vi "SerialComSub.vi"(4 "stop":bool, 6 "input cluster":T1, 7 "state":i64, 9 "Send":bool, 10 "Bool Refnum":refnum<vi>, 11 "VISA Refnum in":refnum<visa-resource-name>) -> (1 "read buffer":string, 2 "return count":u32, 3 "Send return count":u32)   [LabVIEW 2022 SP3]
uses:
  <vilib>/Instr/_visa.llb/VISA Configure Serial Port (Instr).vi
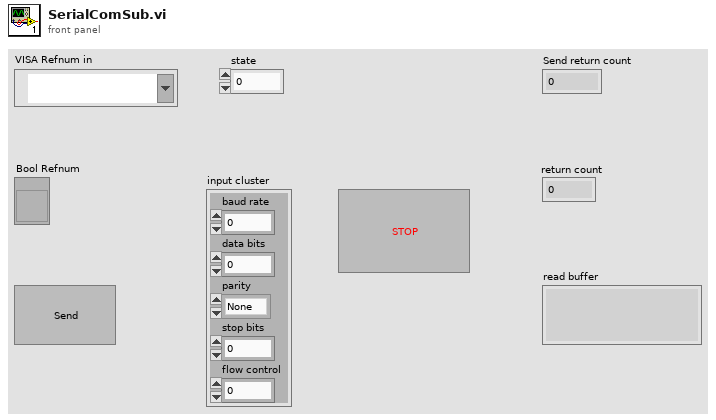
[diagram p1: front panel]
types:
  T1 = cluster{"baud rate":u32, "data bits":u16, "parity":enum16{"None", "Odd", "Even", "Mark", "Space"}, "stop bits":u16, "flow control":u16}
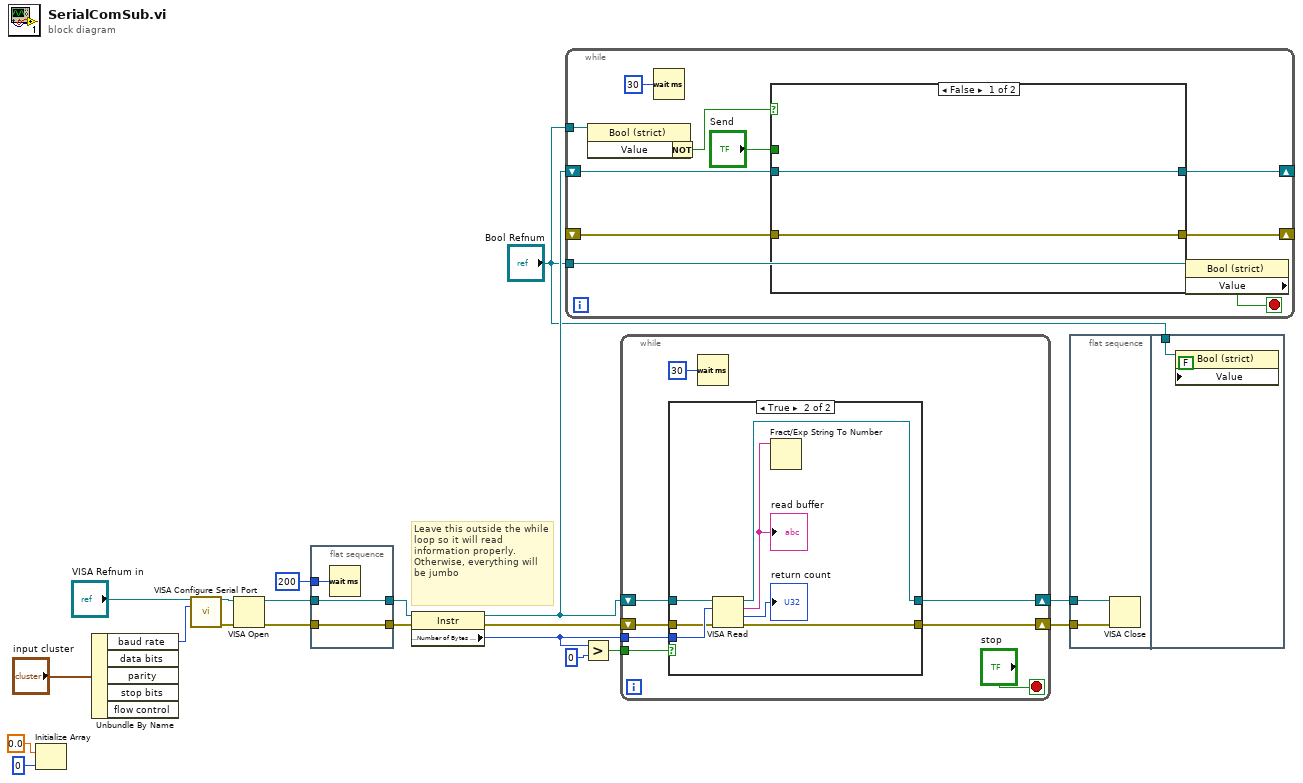
[diagram p0: block diagram]
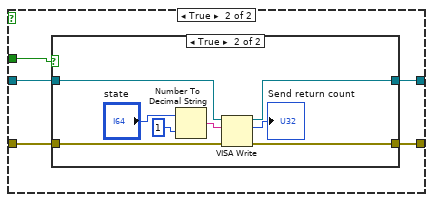
[diagram p2: hidden frame]
diagram:
  # "Leave this outside the while loop so it will read information properly. Otherwise, everything will be jumbo"
  n1 = Initialize Array(0.0, 0) -> ()  [unwired: 1 out]
  n2 = Unbundle By Name("input cluster") -> ("baud rate"=w16:u32)  [unwired: 4 out]
  n3 = call-poly "VISA Configure Serial Port"("VISA resource name"="VISA Refnum in", "baud rate (9600)"=w16) -> ("VISA resource name out"=w18:refnum<visa-resource-name>, "error out"=w19:errorcluster)  [unwired: 12 in]
  n4 = VISA Open(error in (no error)=w19, VISA resource name=w18) -> (VISA resource name=w3:refnum<visa-resource-name>, error out=w4:errorcluster)  [unwired: 3 in]
  n5 = flat-sequence {
    tunnel: w4 -> [w22]
    tunnel: [w22] -> w20
    tunnel: w3 -> [w21]
    tunnel: [w21] -> w7
    tunnel: u32 200 -> [w23]
    frame #0 {
      n6 = Wait (ms)(milliseconds to wait=w23) -> ()  [unwired: 1 out]
    }
  }
  n7 = property class="Instr"(reference=w7, error in=w20) -> (reference out=w9:refnum<visa-resource-name>, error out=w11:errorcluster, "Serial Settings:Number of Bytes at Serial Port"=w10:u32)
  n8 = while {
    shift-right: [w33] -> _
    shift-left: w9 -> [w34]
    shift-right: [w30] -> _
    shift-left: _ -> [w31]
    tunnel: "Bool Refnum" -> [w25]
    tunnel: "Bool Refnum" -> [w24]
    stop <- w29 stop-if-true
    n9 = property on="Property Node" class="Bool (strict)"(reference=w24) -> ("Value"=w28:bool)  [unwired: 1 in, 2 out]
    n10 = Wait (ms)(milliseconds to wait=u32 30) -> ()  [unwired: 1 out]
    n11 = Not(x=w28) -> (.not. x?=w27:bool)
    n12 = case shown="False" w27 {
      tunnel: w34 -> [w36 w40]
      tunnel: [w36 w37] -> w33
      tunnel: w31 -> [w35 w39]
      tunnel: [w35 w38] -> w30
      tunnel: "Send" -> [_ w41]
      frame False {
      }
      frame True {
        n13 = case shown="True" w41 {
          tunnel: w40 -> [w43 w47]
          tunnel: w39 -> [w42 w46]
          tunnel: [w42 w44] -> w38
          tunnel: [w43 w45] -> w37
          frame False {
          }
          frame True {
            n14 = Number To Decimal String(number="state", width (-)=i16 1) -> (decimal integer string=w50:string)
            n15 = VISA Write(VISA resource name=w47, write buffer=w50, error in (no error)=w46) -> (VISA resource name out=w45:refnum<visa-resource-name>, return count=→"Send return count":u32, error out=w44:errorcluster)
          }
        }
      }
    }
    n16 = property on="Property Node" class="Bool (strict)"(reference=w25) -> ("Value"=w29:bool)  [unwired: 1 in, 2 out]
  }
  n17 = Greater?(x=w10, y=u32 0) -> (0:w8:bool)
  n18 = while {
    shift-right: [w54] -> w12
    shift-left: w11 -> [w55]
    tunnel: w8 -> [w59]
    tunnel: w10 -> [w58]
    shift-right: [w57] -> w13
    shift-left: w9 -> [w56]
    stop <- "stop" stop-if-true
    n19 = case shown="True" w59 {
      tunnel: w56 -> [w61 w67]
      tunnel: [w61 w66] -> w57
      tunnel: w58 -> [_ w65]
      tunnel: w55 -> [w60 w64]
      tunnel: [w60 w63] -> w54
      frame False {
      }
      frame True {
        n20 = VISA Read(VISA resource name=w67, byte count=w65, error in (no error)=w64) -> (VISA resource name out=w66:refnum<visa-resource-name>, read buffer=w62:string, return count=→"return count":u32, error out=w63:errorcluster)
        "read buffer" <- w62
        n21 = Fract/Exp String To Number(string=w62) -> ()  [unwired: 3 in, 2 out]
      }
    }
    n22 = Wait (ms)(milliseconds to wait=u32 30) -> ()  [unwired: 1 out]
  }
  n23 = flat-sequence {
    tunnel: w12 -> [w70]
    tunnel: w13 -> [w69]
    tunnel: "Bool Refnum" -> [w71]
    frame #0 {
      n24 = VISA Close(VISA resource name=w69, error in (no error)=w70) -> ()  [unwired: 1 out]
    }
    frame #1 {
      n25 = property class="Bool (strict)"(reference=w71, "Value"=FALSE) -> ()  [unwired: 1 in, 2 out]
    }
  }
